vi "Plugin.Set Transceiver Threads.vi"(10 "Transceiver Threads":refnum<class "Transceiver Interface.lvclass">[](array[class]), 11 "Plugin in":refnum<class "Plugin.lvclass">) -> (3 "Plugin out":refnum<class "Plugin.lvclass">)   [LabVIEW 2017, in "DSF Core.lvlib" / "Plugin.lvclass"]
uses:
  Plugin.lvclass
  Interface/Transceiver Interface.lvclass
  Plugin.lvclass/Plugin.ctl
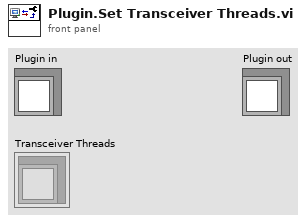
[diagram p1: front panel]
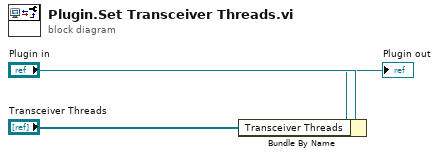
[diagram p0: block diagram]
diagram:
  n1 = Bundle By Name(cluster="Plugin in", "Transceiver Threads"="Transceiver Threads") -> (→"Plugin out":refnum<class "Plugin.lvclass">)
